vi "Fpga-MIX_COL-Top.vi"(10 "Array in":u8[](array[numeric])=[0, 0, 0, 0, 0, 0, 0, 0, 0, 0, 0, 0, 0, 0, 0, 0], 11 "index":i32) -> (3 "Array out":u8[](array[numeric]))   [LabVIEW 2017]
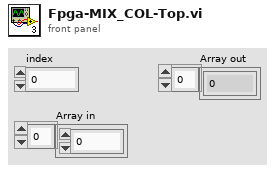
[diagram p1: front panel]
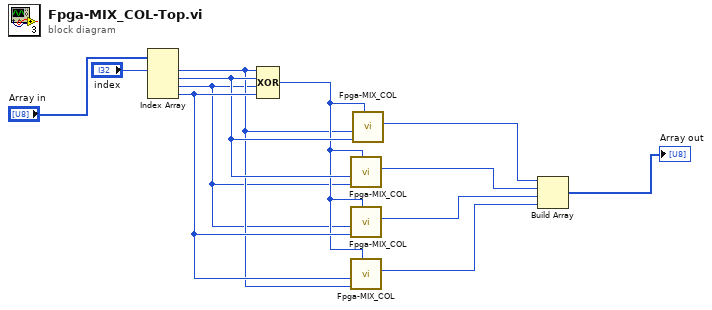
[diagram p0: block diagram]
diagram:
  n1 = Index Array(array="Array in", index #1="index") -> (element #1=w2:u8, element #2=w8:u8, element #3=w1:u8, element #4=w9:u8)  [unwired: 3 in]
  n2 = Compound Arithmetic op=XOR(w2, w8, w1, w9) -> (w7:u8)
  n3 = call "Fpga-MIX_COL.vi"("Tmp"=w7, "state[i][y]"=w1, "state[i][x]"=w8) -> ("state[i][x]"=w10:u8)  [unwired: 8 in]
  n4 = call "Fpga-MIX_COL.vi"("Tmp"=w7, "state[i][y]"=w9, "state[i][x]"=w1) -> ("state[i][x]"=w11:u8)  [unwired: 8 in]
  n5 = call "Fpga-MIX_COL.vi"("Tmp"=w7, "state[i][y]"=w2, "state[i][x]"=w9) -> ("state[i][x]"=w12:u8)  [unwired: 8 in]
  n6 = call "Fpga-MIX_COL.vi"("Tmp"=w7, "state[i][y]"=w8, "state[i][x]"=w2) -> ("state[i][x]"=w6:u8)  [unwired: 8 in]
  n7 = Build Array(w6, w10, w11, w12) -> (→"Array out":u8[])
